vi "Get Array.vi"(8 "error in (no error)":errorcluster, 10 "Name Array":string[](array[string]), 11 "JSON Array in":refnum<class "JSON Value.lvclass">) -> (0 "error out":errorcluster, 2 "Array":refnum<class "JSON Value.lvclass">[](array[class]), 3 "JSON Array out":refnum<class "JSON Value.lvclass">)   [LabVIEW 2011, in "JSON Array.lvclass"]
uses:
  JSON Array.lvclass
  JSON Value/JSON Value.lvclass
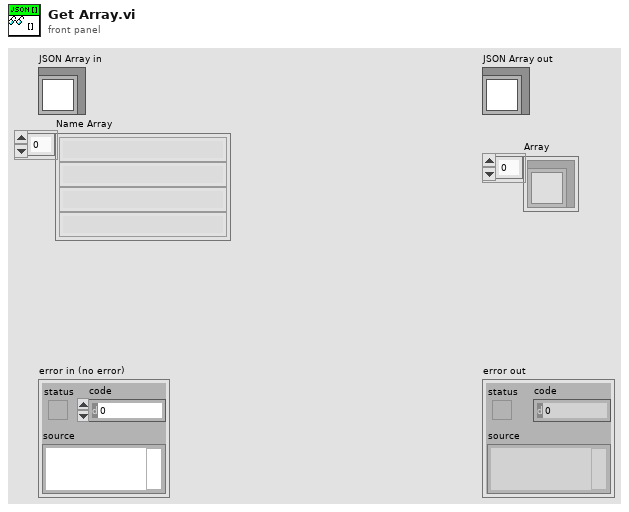
[diagram p1: front panel]
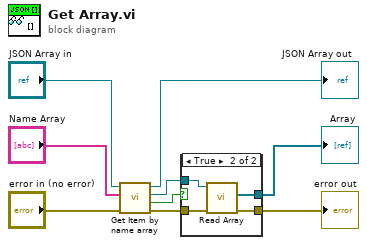
[diagram p0: block diagram]
diagram:
  n1 = call "Get Item by name array.vi"("error in (no error)"="error in (no error)", "Name Array"="Name Array", "JSON Value In"="JSON Array in") -> ("error out"=w9:errorcluster, "found"=w8:bool, "Value"=w7:refnum<class "JSON Value.lvclass">, "JSON Value Out"=→"JSON Array out":refnum<class "JSON Value.lvclass">)  [unwired: 5 in]
  n2 = case shown="True" w8 {
    tunnel: w7 -> [_ w14]
    tunnel: [_ w13] -> w4
    tunnel: w9 -> [w10 w12]
    tunnel: [w10 w11] -> w3
    frame False {
    }
    frame True {
      n3 = call-dynamic "Read Array.vi"("error in (no error)"=w12, "JSON Value In"=w14) -> ("error out"=w11:errorcluster, "Array"=w13:refnum<class "JSON Value.lvclass">[])  [unwired: 7 in, 1 out]
    }
  }
  "error out" <- w3
  "Array" <- w4
